vi "dev-cmd-struct-add-info.vi"(10 "info":T3, 11 "dev-cmd":T1) -> (3 "dev-cmd out":T1)   [LabVIEW 2019]
panel:
  out "cmd":string
  in  "device":T2
  in  "组合框":string(combo)
  in  "device-list out":T4(array[cluster])
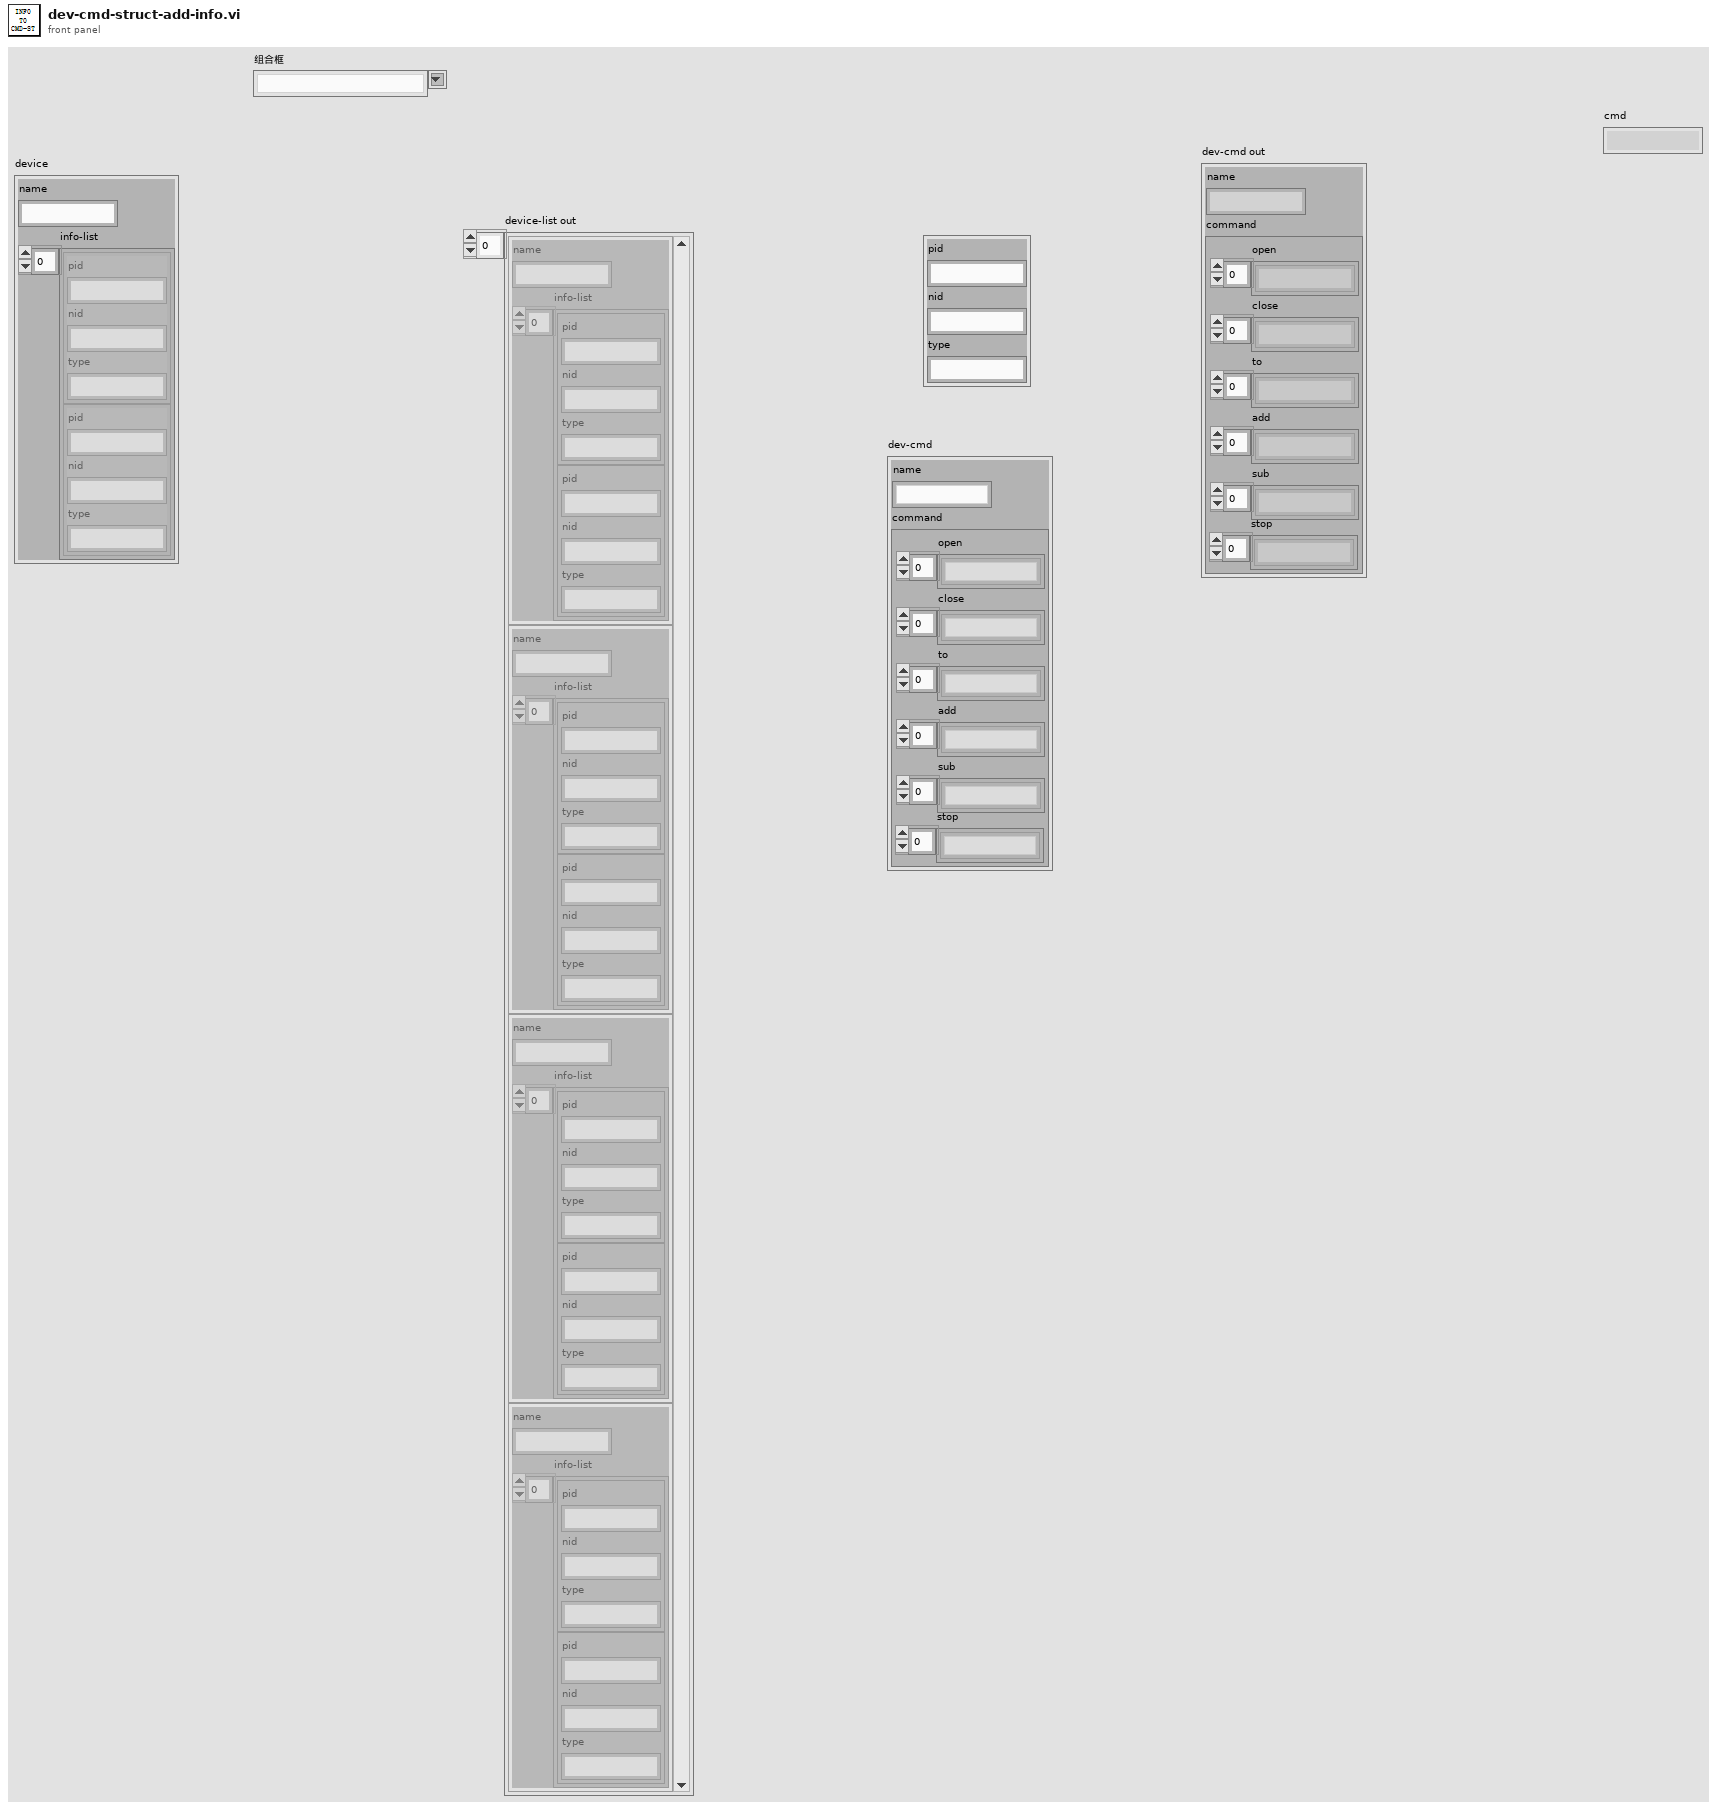
[diagram p1: front panel]
types:
  T1 = cluster{"command":cluster{"open":string[], "close":string[], "to":string[], "add":string[], "sub":string[], "stop":string[]}, "name":string}
  T2 = cluster{"name":string, "info-list":cluster{"pid":string, "nid":string, "type":string}[]}
  T3 = cluster{"pid":string, "nid":string, "type":string}
  T4 = cluster{"name":string, "info-list":cluster{"pid":string, "nid":string, "type":string}[]}[]
  T5 = enum16{"open", "close", "to", "add", "sub", "stop"}
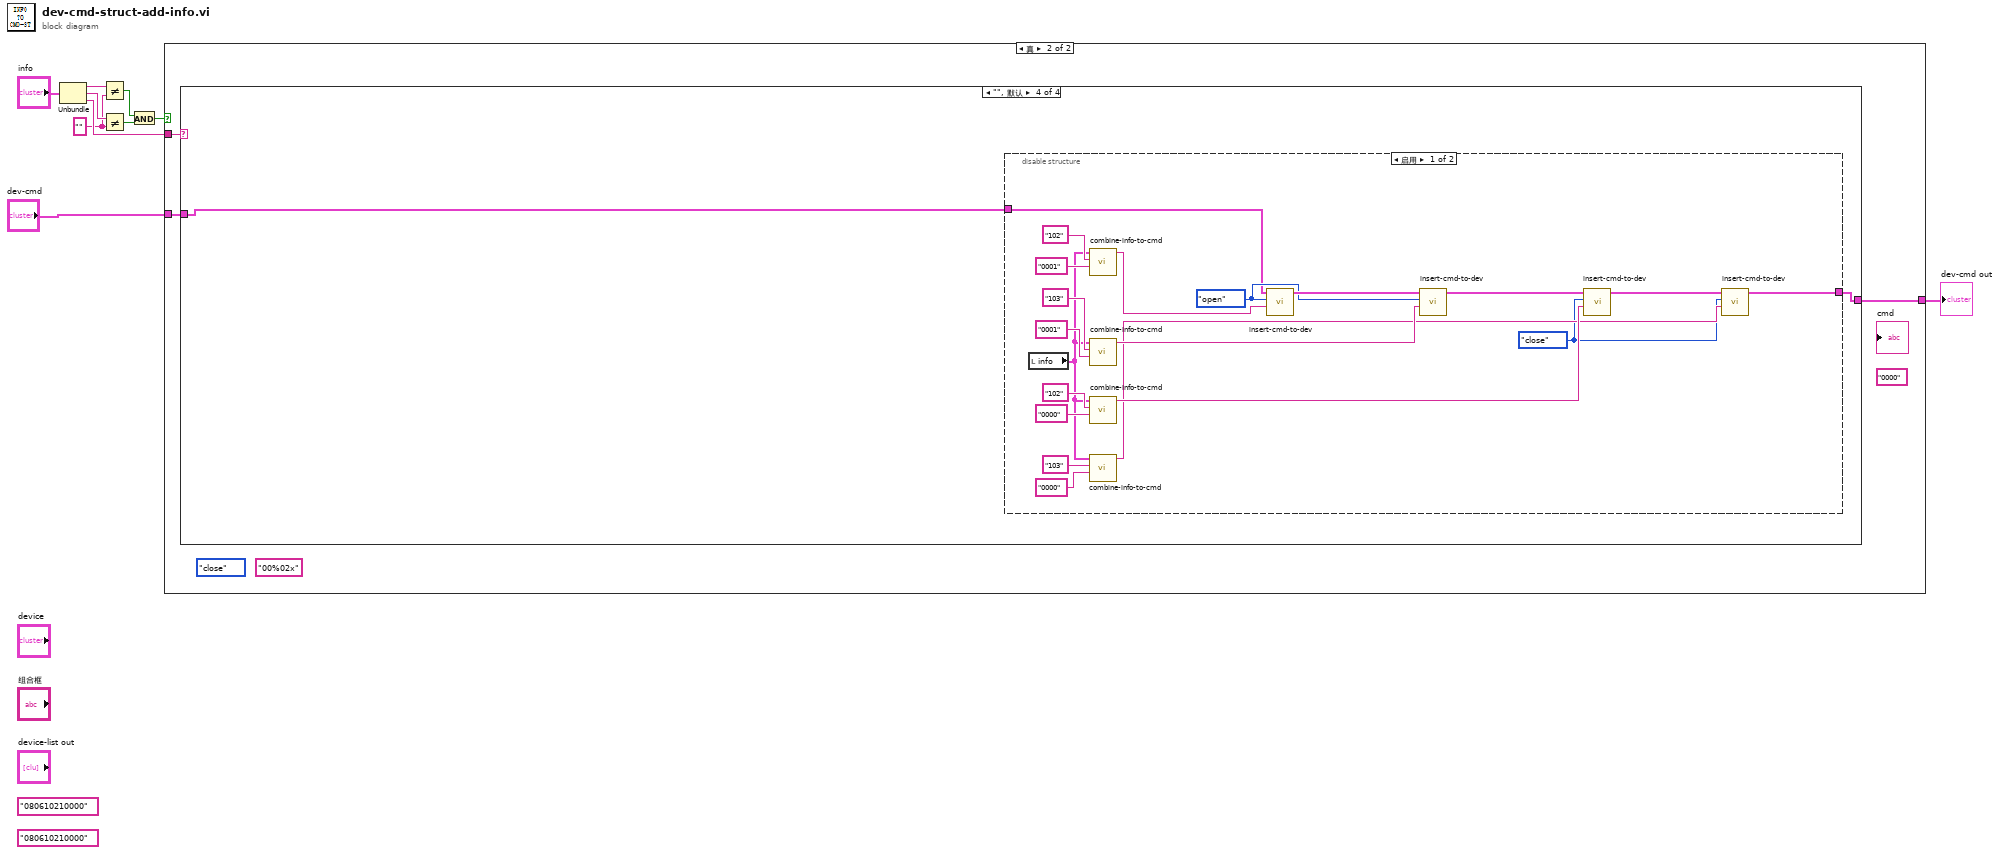
[diagram p0: block diagram]
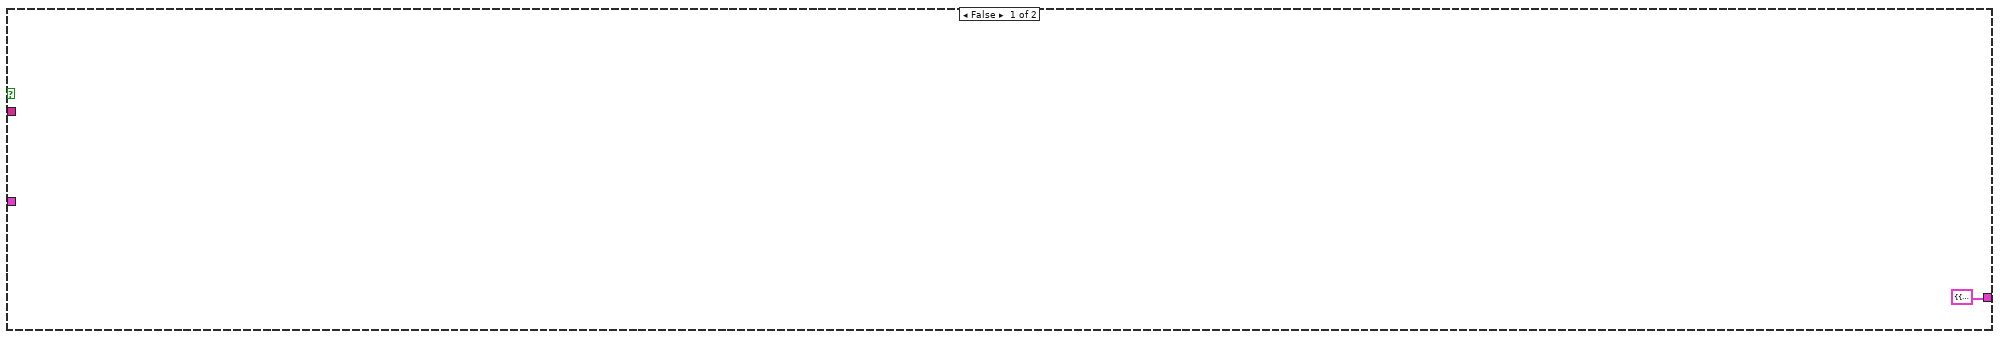
[diagram p2: hidden frame]
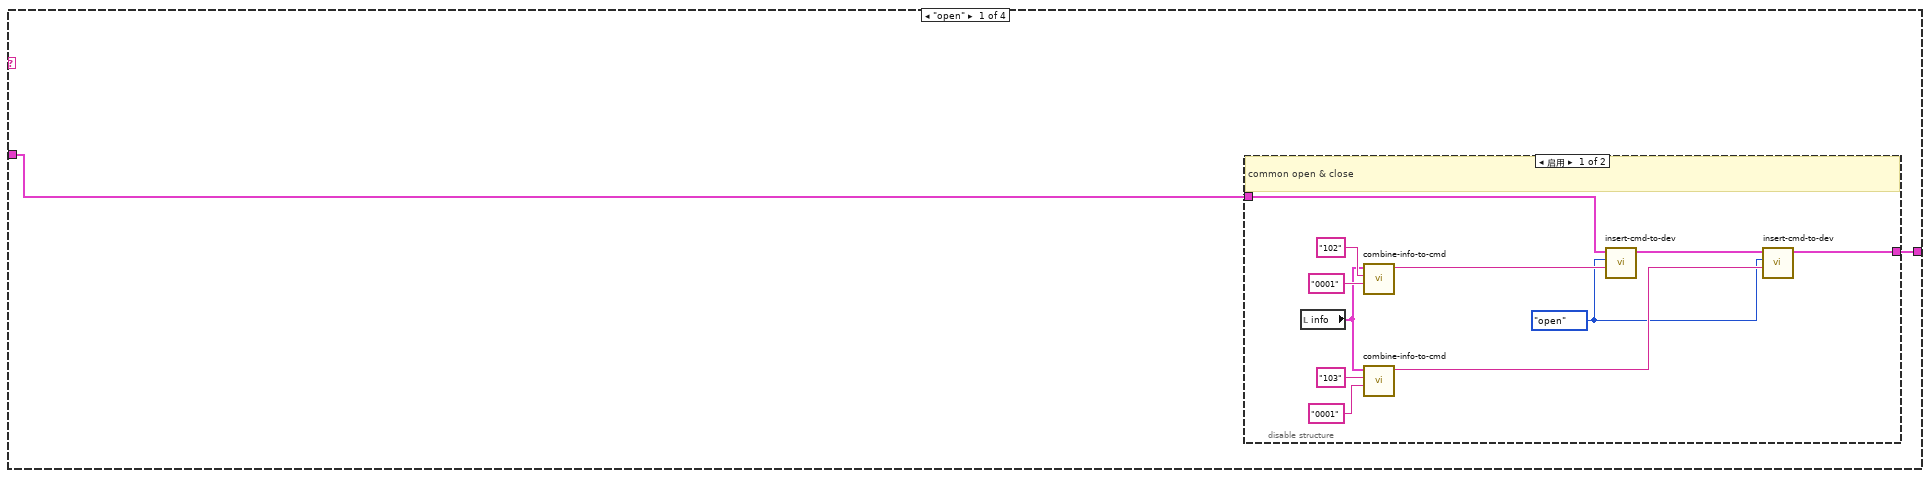
[diagram p3: hidden frame]
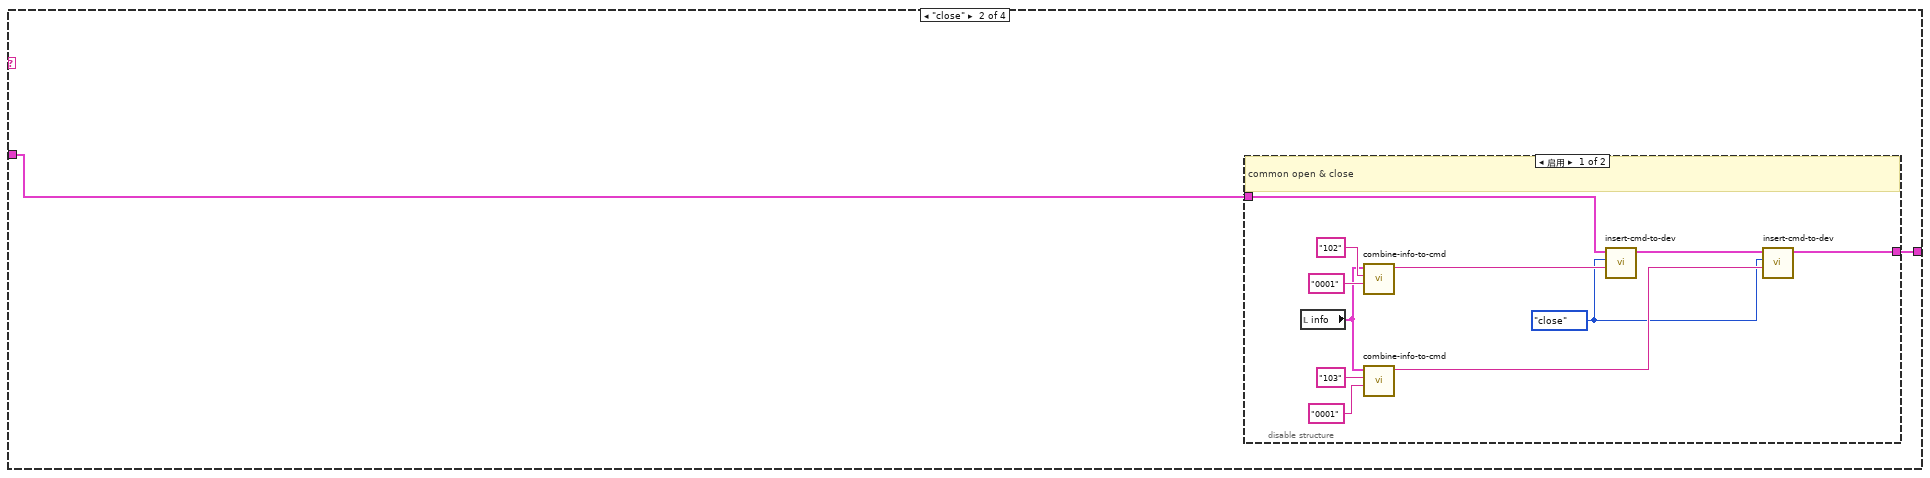
[diagram p5: hidden frame]
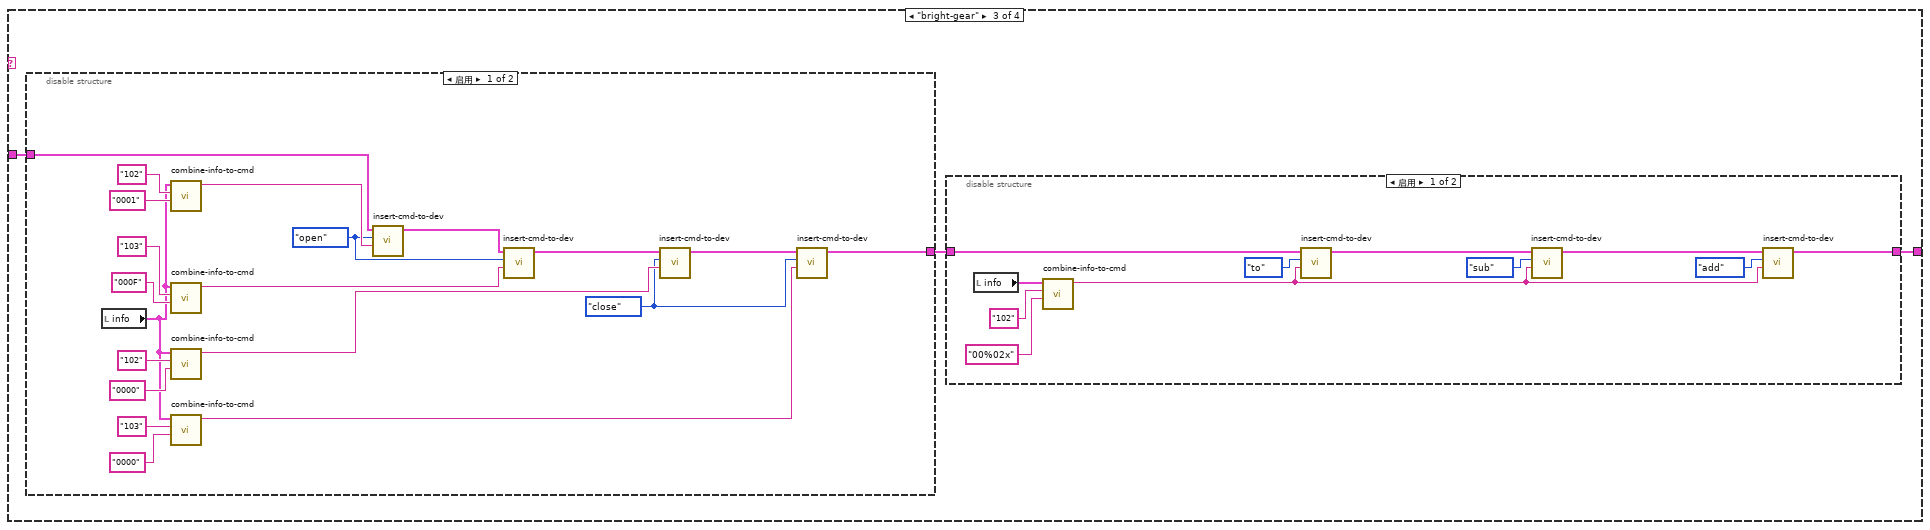
[diagram p7: hidden frame]
diagram:
  w6 = "" ("y")
  (unwired) "080610210000" ("字符串")
  (unwired) "080610210000" ("字符串")
  n1 = Unbundle("info") -> ("pid"=w8:string, "nid"=w7:string, "type"=w9:string)
  n2 = Not Equal?(x=w8, y=w6) -> (x != y?=w2:bool)
  n3 = Not Equal?(x=w7, y=w6) -> (x != y?=w3:bool)
  n4 = And(x=w2, y=w3) -> (x .and. y?=w4:bool)
  n5 = case shown="真" w4 {
    tunnel: w9 -> [_ w14]
    tunnel: [T1 {"command"={"open"=[], "close"=[], "to"=[], "add"=[], "sub"=[], "stop"=[]}, "name"=""} ("dev-cmd out") w13] -> w5
    tunnel: "dev-cmd" -> [_ w12]
    frame False {
    }
    frame True {
      (unwired) T5."close" ("枚举")
      (unwired) "0000" ("字符串")
      (unwired) "00%02x" ("字符串")
      n6 = case shown="\"\", 默认" w14 {
        tunnel: [w16 w29 w42 w76] -> w13
        tunnel: w12 -> [w15 w28 w41 w75]
        frame "open" {
          n7 = disable-structure shown="启用" {
            disable-tunnel: [w19 _] -> w16
            disable-tunnel: w15 -> [w17 _]
            frame Enabled {
              w18 = T5."open" ("枚举")
              # "common open & close"
              n8 = local read "info"() -> (w20:T3)
              n9 = call "combine-info-to-cmd.vi"("值"="0001" ("字符串"), "寄存器"="102" ("字符串"), "info"=w20) -> ("command"=w24:string)  [unwired: 8 in]
              n10 = call "combine-info-to-cmd.vi"("值"="0001" ("字符串"), "寄存器"="103" ("字符串"), "info"=w20) -> ("command"=w21:string)  [unwired: 8 in]
              n11 = call "insert-cmd-to-dev.vi"("字符串"=w24, "枚举"=w18, "dev-cmd"=w17) -> ("dev-cmd out"=w27:T1)  [unwired: 8 in]
              n12 = call "insert-cmd-to-dev.vi"("字符串"=w21, "枚举"=w18, "dev-cmd"=w27) -> ("dev-cmd out"=w19:T1)  [unwired: 8 in]
            }
            frame Disabled {
            }
          }
        }
        frame "close" {
          n13 = disable-structure shown="启用" {
            disable-tunnel: [w32 _] -> w29
            disable-tunnel: w28 -> [w30 _]
            frame Enabled {
              w31 = T5."close" ("枚举")
              # "common open & close"
              n14 = local read "info"() -> (w33:T3)
              n15 = call "combine-info-to-cmd.vi"("值"="0001" ("字符串"), "寄存器"="102" ("字符串"), "info"=w33) -> ("command"=w37:string)  [unwired: 8 in]
              n16 = call "combine-info-to-cmd.vi"("值"="0001" ("字符串"), "寄存器"="103" ("字符串"), "info"=w33) -> ("command"=w34:string)  [unwired: 8 in]
              n17 = call "insert-cmd-to-dev.vi"("字符串"=w37, "枚举"=w31, "dev-cmd"=w30) -> ("dev-cmd out"=w40:T1)  [unwired: 8 in]
              n18 = call "insert-cmd-to-dev.vi"("字符串"=w34, "枚举"=w31, "dev-cmd"=w40) -> ("dev-cmd out"=w32:T1)  [unwired: 8 in]
            }
            frame Disabled {
            }
          }
        }
        frame "bright-gear" {
          n19 = disable-structure shown="启用" {
            disable-tunnel: [w65 _] -> w43
            disable-tunnel: w41 -> [w55 _]
            frame Enabled {
              w56 = T5."close" ("枚举")
              w57 = T5."open" ("枚举")
              n20 = local read "info"() -> (w58:T3)
              n21 = call "combine-info-to-cmd.vi"("值"="0001" ("字符串"), "寄存器"="102" ("字符串"), "info"=w58) -> ("command"=w71:string)  [unwired: 8 in]
              n22 = call "combine-info-to-cmd.vi"("值"="000F" ("字符串"), "寄存器"="103" ("字符串"), "info"=w58) -> ("command"=w68:string)  [unwired: 8 in]
              n23 = call "combine-info-to-cmd.vi"("值"="0000" ("字符串"), "寄存器"="102" ("字符串"), "info"=w58) -> ("command"=w60:string)  [unwired: 8 in]
              n24 = call "combine-info-to-cmd.vi"("值"="0000" ("字符串"), "寄存器"="103" ("字符串"), "info"=w58) -> ("command"=w59:string)  [unwired: 8 in]
              n25 = call "insert-cmd-to-dev.vi"("字符串"=w71, "枚举"=w57, "dev-cmd"=w55) -> ("dev-cmd out"=w74:T1)  [unwired: 8 in]
              n26 = call "insert-cmd-to-dev.vi"("字符串"=w68, "枚举"=w57, "dev-cmd"=w74) -> ("dev-cmd out"=w66:T1)  [unwired: 8 in]
              n27 = call "insert-cmd-to-dev.vi"("字符串"=w60, "枚举"=w56, "dev-cmd"=w66) -> ("dev-cmd out"=w67:T1)  [unwired: 8 in]
              n28 = call "insert-cmd-to-dev.vi"("字符串"=w59, "枚举"=w56, "dev-cmd"=w67) -> ("dev-cmd out"=w65:T1)  [unwired: 8 in]
            }
            frame Disabled {
            }
          }
          n29 = disable-structure shown="启用" {
            disable-tunnel: [w48 _] -> w42
            disable-tunnel: w43 -> [w47 _]
            frame Enabled {
              n30 = local read "info"() -> (w50:T3)
              n31 = call "combine-info-to-cmd.vi"("值"="00%02x" ("字符串"), "寄存器"="102" ("字符串"), "info"=w50) -> ("command"=w49:string)  [unwired: 8 in]
              n32 = call "insert-cmd-to-dev.vi"("字符串"=w49, "枚举"=T5."to", "dev-cmd"=w47) -> ("dev-cmd out"=w54:T1)  [unwired: 8 in]
              n33 = call "insert-cmd-to-dev.vi"("字符串"=w49, "枚举"=T5."sub", "dev-cmd"=w54) -> ("dev-cmd out"=w51:T1)  [unwired: 8 in]
              n34 = call "insert-cmd-to-dev.vi"("字符串"=w49, "枚举"=T5."add", "dev-cmd"=w51) -> ("dev-cmd out"=w48:T1)  [unwired: 8 in]
            }
            frame Disabled {
            }
          }
        }
        frame "", Default {
          n35 = disable-structure shown="启用" {
            disable-tunnel: [w80 _] -> w76
            disable-tunnel: w75 -> [w77 _]
            frame Enabled {
              w78 = T5."close" ("枚举")
              w79 = T5."open" ("枚举")
              n36 = local read "info"() -> (w81:T3)
              n37 = call "combine-info-to-cmd.vi"("值"="0001" ("字符串"), "寄存器"="102" ("字符串"), "info"=w81) -> ("command"=w93:string)  [unwired: 8 in]
              n38 = call "combine-info-to-cmd.vi"("值"="0001" ("字符串"), "寄存器"="103" ("字符串"), "info"=w81) -> ("command"=w90:string)  [unwired: 8 in]
              n39 = call "combine-info-to-cmd.vi"("值"="0000" ("字符串"), "寄存器"="102" ("字符串"), "info"=w81) -> ("command"=w83:string)  [unwired: 8 in]
              n40 = call "combine-info-to-cmd.vi"("值"="0000" ("字符串"), "寄存器"="103" ("字符串"), "info"=w81) -> ("command"=w82:string)  [unwired: 8 in]
              n41 = call "insert-cmd-to-dev.vi"("字符串"=w93, "枚举"=w79, "dev-cmd"=w77) -> ("dev-cmd out"=w96:T1)  [unwired: 8 in]
              n42 = call "insert-cmd-to-dev.vi"("字符串"=w90, "枚举"=w79, "dev-cmd"=w96) -> ("dev-cmd out"=w88:T1)  [unwired: 8 in]
              n43 = call "insert-cmd-to-dev.vi"("字符串"=w83, "枚举"=w78, "dev-cmd"=w88) -> ("dev-cmd out"=w89:T1)  [unwired: 8 in]
              n44 = call "insert-cmd-to-dev.vi"("字符串"=w82, "枚举"=w78, "dev-cmd"=w89) -> ("dev-cmd out"=w80:T1)  [unwired: 8 in]
            }
            frame Disabled {
            }
          }
        }
      }
    }
  }
  "dev-cmd out" <- w5
